vi "Write Write_.vi"(8 "error in (no error)":errorcluster, 10 "Write?":bool, 11 "Set Wvfm Write CMD in":refnum<class "Set Wvfm Write CMD.lvclass">) -> (0 "error out":errorcluster, 3 "Set Wvfm Write CMD out":refnum<class "Set Wvfm Write CMD.lvclass">)   [LabVIEW 2014, in "ePAS Library.lvlib" / "Set Wvfm Write CMD.lvclass"]
uses:
  Set Wvfm Write CMD.lvclass
  Set Wvfm Write CMD.lvclass/Set Wvfm Write CMD.ctl
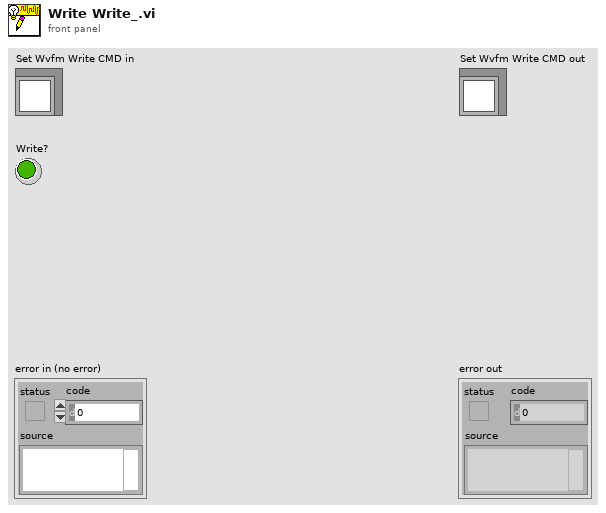
[diagram p1: front panel]
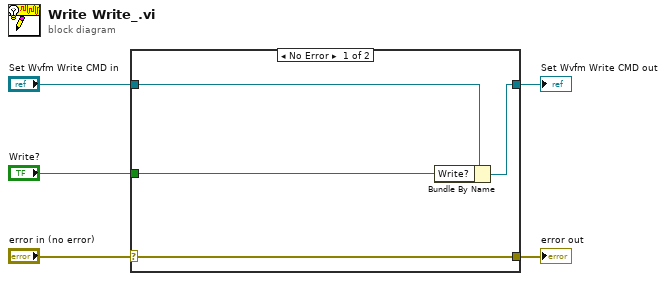
[diagram p0: block diagram]
diagram:
  n1 = case shown="No Error" "error in (no error)" {
    selector: "error in (no error)" -> [w9 w10]
    tunnel: [w9 w10] -> w4
    tunnel: [w7 w11] -> w2
    tunnel: "Set Wvfm Write CMD in" -> [w8 w11]
    tunnel: "Write?" -> [w6 _]
    frame No Error {
      n2 = Bundle By Name(cluster=w8, "Write?"=w6) -> (w7:refnum<class "Set Wvfm Write CMD.lvclass">)
    }
    frame Error {
    }
  }
  "error out" <- w4
  "Set Wvfm Write CMD out" <- w2
